vi "Power On (uSMC).vi"(8 "error in (no error)":errorcluster, 9 "Index":i32, 11 "Visa Array in":refnum<visa-resource-name>[](array[refnum])) -> (0 "error out":errorcluster, 3 "Visa Array out":refnum<visa-resource-name>[](array[refnum]))   [LabVIEW 2010, in "SignalWriterMH110203USBStepperMotor.lvclass"]
uses:
  SignalWriterMH110203USBStepperMotor.lvclass
  class_data.vi
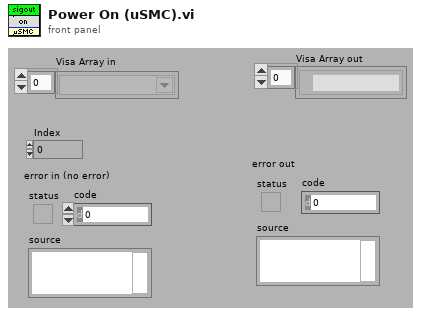
[diagram p1: front panel]
types:
  T1 = typedef "SignalWriterMH110203USBStepperMotor.lvclass/Mode Control (uSMC).ctl" = cluster{"Turn Buttons Off":bool, "Reduce Current":bool, "Power Off and Make a Whole Step":bool, "Emergency Power Off":bool, "Limit Switch 1 True State":bool, "Limit Switch 2 True State":bool, "Rotary Transducer TRUE State":bool, "Swap Limit Switches":bool, "Limit Switch 1 Operation Enabled":bool, "Limit Switch 2 Operation Enabled":bool, "Rotary Transducer Operation Enabled":bool, "Rotary Transducer Operation Select":bool, "Button 1 True State":bool, "Button 2 True State":bool, "Swap Buttons":bool, "Reset Rotary Transducer Check Positions":bool, "Output Syncronization Enabled":bool, "Reset Output Sync Count":bool, "Sync Operation":bool, "Sync Count":u32, "Power":bool, "Invert Sync Polarity":bool, "Use Encoder":bool, "Invert Encoder Direction":bool, "Reset Encoder To 0":bool, "Reset SM Enc Pos to Enc Pos":bool}
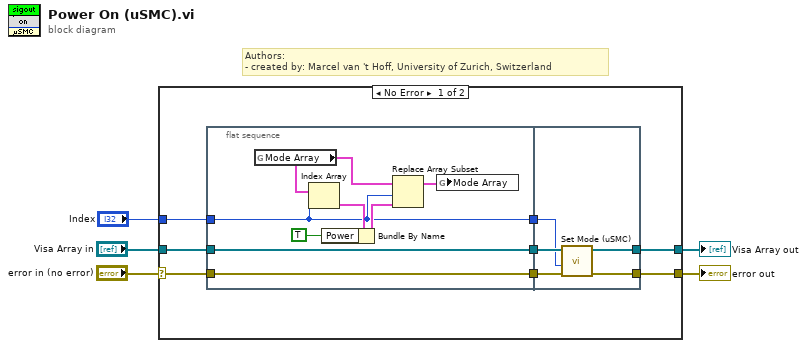
[diagram p0: block diagram]
diagram:
  # "Authors: \n- created by: Marcel van 't Hoff, University of Zurich, Switzerland"
  n1 = case shown="No Error" "error in (no error)" {
    selector: "error in (no error)" -> [w7 w27]
    tunnel: "Visa Array in" -> [w10 w28]
    tunnel: [w9 w28] -> w4
    tunnel: [w8 w27] -> w3
    tunnel: "Index" -> [w6 _]
    frame No Error {
      n2 = flat-sequence {
        tunnel: w10 -> [w17]
        tunnel: [w17] -> w13
        tunnel: [w16] -> w12
        tunnel: w7 -> [w16]
        tunnel: [w14] -> w11
        tunnel: w6 -> [w14]
        tunnel: w13 -> [w26]
        tunnel: w12 -> [w25]
        tunnel: w11 -> [w24]
        tunnel: [w23] -> w9
        tunnel: [w22] -> w8
        frame #0 {
          n3 = global read "class_data.vi" "Mode Array"() -> (w19:T1[])
          n4 = Index Array(array=w19, index=w14) -> (element=w21:T1)
          n5 = Bundle By Name(cluster=w21, "Power"=TRUE ("emergency power off")) -> (w18:T1)
          n6 = Replace Array Subset(array=w19, new element=w18, index=w14) -> (w15:T1[])
          n7 = global write "class_data.vi" "Mode Array"(w15) -> ()
        }
        frame #1 {
          n8 = call "Set Mode (uSMC).vi"("error in (no error)"=w25, "Index"=w24, "Visa Array in"=w26) -> ("error out"=w22:errorcluster, "Visa Array out"=w23:refnum<visa-resource-name>[])  [unwired: 7 in]
        }
      }
    }
    frame Error {
    }
  }
  "Visa Array out" <- w4
  "error out" <- w3
